vi "Read Open_Close.vi"(8 "error in (no error)":errorcluster, 11 "PacMan in":refnum<class "PacMan.lvclass">) -> (0 "error out":errorcluster, 2 "Open/Close":bool, 3 "PacMan out":refnum<class "PacMan.lvclass">)   [LabVIEW 2016, in "PacManClasses.lvlib" / "PacMan.lvclass"]
uses:
  PacMan.lvclass
  PacMan.lvclass/PacMan.ctl
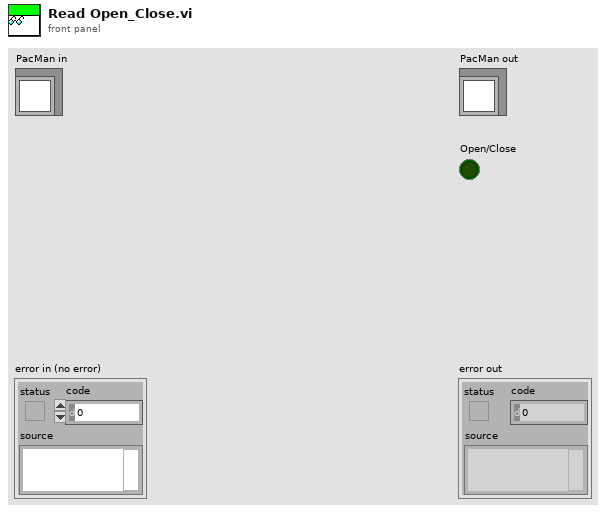
[diagram p1: front panel]
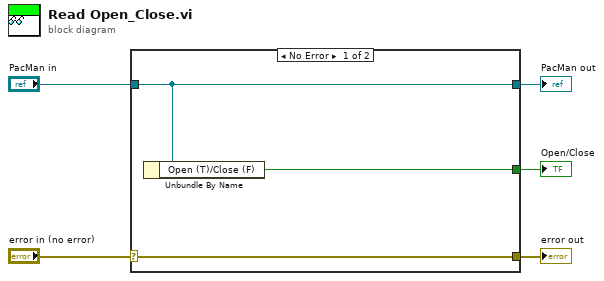
[diagram p0: block diagram]
diagram:
  n1 = case shown="No Error" "error in (no error)" {
    selector: "error in (no error)" -> [w8 w9]
    tunnel: [w8 w9] -> w4
    tunnel: [w7 w10] -> w2
    tunnel: "PacMan in" -> [w7 w10]
    tunnel: [w6 _] -> w1
    frame No Error {
      n2 = Unbundle By Name(w7) -> ("Open (T)/Close (F)"=w6:bool)
    }
    frame Error {
    }
  }
  "error out" <- w4
  "PacMan out" <- w2
  "Open/Close" <- w1
